vi "I.vi"(1 "sum[k-1]":dbl, 2 "Ts":dbl, 3 "error":dbl) -> (0 "sum":dbl)   [LabVIEW 2011]
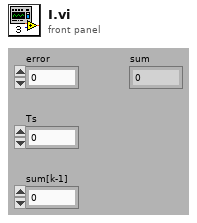
[diagram p1: front panel]
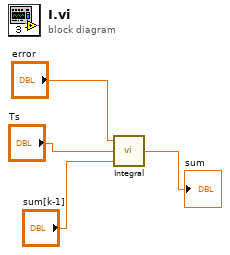
[diagram p0: block diagram]
diagram:
  n1 = call "Integral.vi"("sum[k-1]"="sum[k-1]", "Ts"="Ts", "error"="error") -> ("sum"=→"sum":dbl)
